vi "Display Winner.vi"(11 "Game Board in":refnum<class "Game Board.lvclass">) -> ()   [LabVIEW 2021, in "Game Board.lvclass"]
doc: "MIT Licence\nCopyright (c) 2024 David Grollier"
uses:
  Game Board.lvclass
  Game Board.lvclass/Game Board.ctl
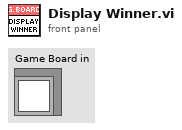
[diagram p1: front panel]
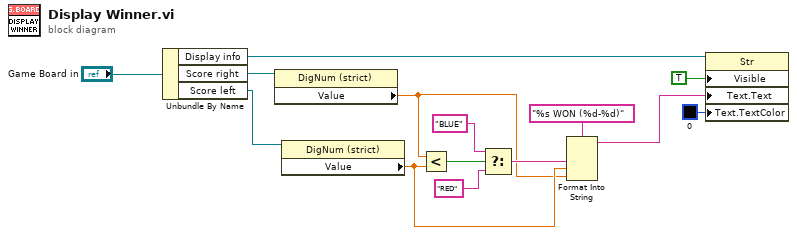
[diagram p0: block diagram]
diagram:
  n1 = Unbundle By Name("Game Board in") -> ("Display info"=w10:refnum<vi>, "Score right"=w14:refnum<vi>, "Score left"=w13:refnum<vi>)
  n2 = property class="DigNum (strict)"(reference=w14) -> ("Value"=w1:dbl)  [unwired: 1 in, 2 out]
  n3 = property class="DigNum (strict)"(reference=w13) -> ("Value"=w2:dbl)  [unwired: 1 in, 2 out]
  n4 = Less?(x=w1, y=w2) -> (x < y?=w8:bool)
  n5 = Select(t="BLUE", s=w8, f="RED") -> (s? t:f=w4:string)
  n6 = Format Into String(format string="%s WON (%d-%d)", w4, w2, w1) -> (resulting string=w3:string)  [unwired: 2 in, 1 out]
  n7 = property class="Str"(reference=w10, "Visible"=TRUE, "Text.Text"=w3, "Text.TextColor"=u32 0 ("Text.Text Colors:Text Color")) -> ()  [unwired: 1 in, 2 out]
